vi "Add Coord (SubVI).vi"(8 "X":bool, 10 "End Point Coordinates in":cluster{"X (m)":sgl, "Y (m)":sgl}, 11 "Numeric":sgl) -> (3 "End Point Coordinates out":cluster{"X (m)":sgl, "Y (m)":sgl})   [LabVIEW 2014]
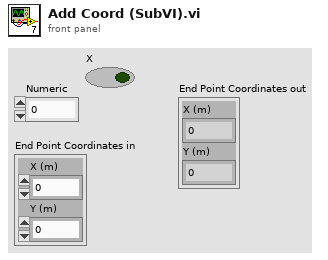
[diagram p1: front panel]
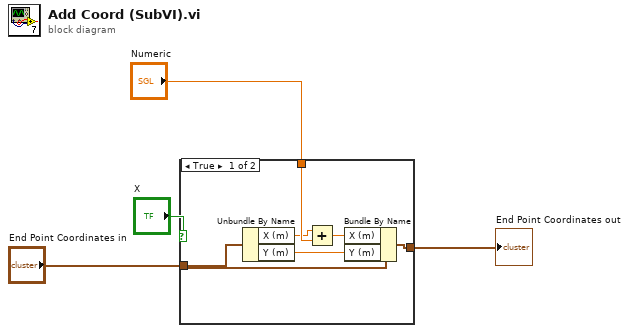
[diagram p0: block diagram]
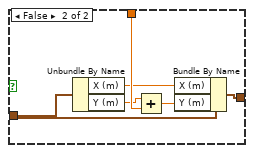
[diagram p2: hidden frame]
diagram:
  n1 = case shown="True" "X" {
    tunnel: [w10 w16] -> w4
    tunnel: "End Point Coordinates in" -> [w9 w15]
    tunnel: "Numeric" -> [w8 w14]
    frame True {
      n2 = Unbundle By Name(w9) -> ("X (m)"=w5:sgl, "Y (m)"=w7:sgl)
      n3 = Add(x=w5, y=w8) -> (x+y=w6:sgl)
      n4 = Bundle By Name(cluster=w9, "X (m)"=w6, "Y (m)"=w7) -> (w10:cluster{"X (m)":sgl, "Y (m)":sgl})
    }
    frame False {
      n5 = Unbundle By Name(w15) -> ("X (m)"=w11:sgl, "Y (m)"=w13:sgl)
      n6 = Add(x=w13, y=w14) -> (x+y=w12:sgl)
      n7 = Bundle By Name(cluster=w15, "X (m)"=w11, "Y (m)"=w12) -> (w16:cluster{"X (m)":sgl, "Y (m)":sgl})
    }
  }
  "End Point Coordinates out" <- w4
